vi "SendEth.vi"(4 "Msg":T1, 5 "conn ID":refnum<k5>) -> (1 "status":bool)   [LabVIEW 2017]
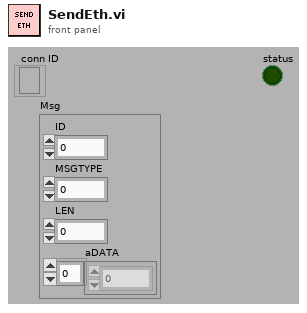
[diagram p1: front panel]
types:
  T1 = cluster{"ID":u32, "MSGTYPE":u8, "LEN":u8, "aDATA":u8[]}
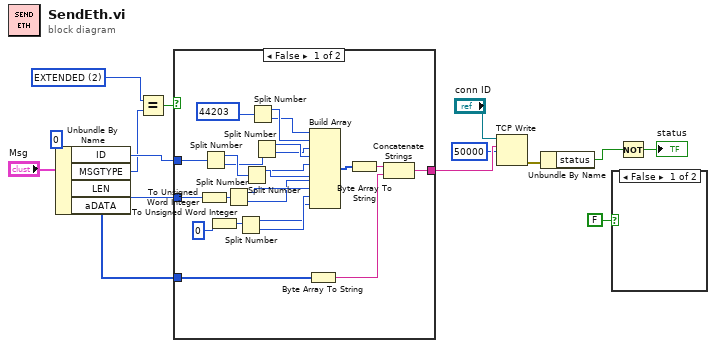
[diagram p0: block diagram]
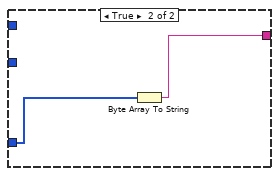
[diagram p2: hidden frame]
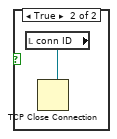
[diagram p3: hidden frame]
diagram:
  w2 = u8 2 items=["STATUS"=128, "EXTENDED"=2, "RTR"=1, "DATA MSG"=0] ("MSGTYPE")
  (unwired) u8 0 ("MSGTYPE")
  n1 = Unbundle By Name("Msg") -> ("ID"=w5:u32, "MSGTYPE"=w1:u8, "LEN"=w9:u8, "aDATA"=w12:u8[])
  n2 = Equal?(x=w2, y=w1) -> (x = y?=w3:bool)
  n3 = case shown="False" w3 {
    tunnel: w12 -> [w37 w39]
    tunnel: [w33 w38] -> w11
    tunnel: w9 -> [w23 _]
    tunnel: w5 -> [w20 _]
    frame False {
      n4 = To Unsigned Word Integer(number=w23) -> (unsigned 16bit integer=w22:u16)
      n5 = Split Number(x=w20) -> (hi(x)=w29:u16, lo(x)=w24:u16)
      n6 = To Unsigned Word Integer(number=u32 0 ("x")) -> (unsigned 16bit integer=w15:u16)
      n7 = Split Number(x=w22) -> (hi(x)=w21:u8, lo(x)=w19:u8)
      n8 = Split Number(x=w15) -> (hi(x)=w17:u8, lo(x)=w18:u8)
      n9 = Split Number(x=w29) -> (hi(x)=w26:u8, lo(x)=w25:u8)
      n10 = Split Number(x=u16 44203 ("element")) -> (hi(x)=w32:u8, lo(x)=w31:u8)
      n11 = Split Number(x=w24) -> (hi(x)=w28:u8, lo(x)=w27:u8)
      n12 = Byte Array To String(unsigned byte array=w37) -> (string=w34:string)
      n13 = Build Array(w31, w32, w27, w28, w25, w26, w19, w21, w18, w17) -> (w36:u8[])
      n14 = Byte Array To String(unsigned byte array=w36) -> (string=w35:string)
      n15 = Concatenate Strings(w35, w34) -> (w33:string)
    }
    frame True {
      n16 = Byte Array To String(unsigned byte array=w39) -> (string=w38:string)
    }
  }
  n17 = TCP Write(connection ID="conn ID", data in=w11, 9:50000 ("timeout ms (25000)")) -> (error out=w13:errorcluster)  [unwired: 1 in, 2 out]
  n18 = Unbundle By Name(w13) -> ("status"=w8:bool)
  n19 = case shown="False" FALSE {
    frame False {
    }
    frame True {
      n20 = local read "conn ID"() -> (w40:refnum<k5>)
      n21 = TCP Close Connection(connection ID=w40) -> ()  [unwired: 2 in, 2 out]
    }
  }
  n22 = Not(x=w8) -> (.not. x?=→"status":bool)
